vi "PCO_RecorderCopyAverageImage.vi"(0 "phRec":u64, 1 "wRoiX0":u16, 2 "wRoiX1":u16, 5 "phCam":u64, 7 "dwStartIdx":u32, 9 "dwStopIdx":u32, 11 "error in (no error)":errorcluster {"code" format="%x"}, 12 "wRoiY0":u16, 13 "wRoiY1":u16) -> (4 "phRec out":u64, 6 "ErrorMessage":i32 format="%x", 8 "wImgBuf":u16[][](array[numeric]), 15 "error out":errorcluster {"code" format="%x"})   [LabVIEW 2020, in "Recorder.lvlib"]
doc: "int WINAPI PCO_RecorderCopyAverageImage(HANDLE phRec, HANDLE phCam, DWORD dwStartIdx, DWORD dwStopIdx, WORD wRoiX0, WORD wRoiY0, WORD wRoiX1, WORD wRoiY1, WORD* wImgBuf);"
uses:
  Recorder.lvlib
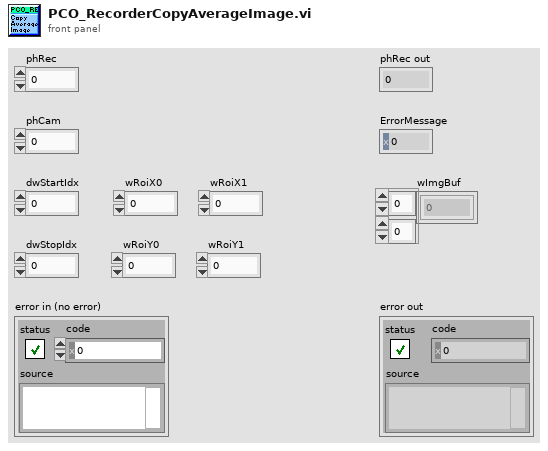
[diagram p1: front panel]
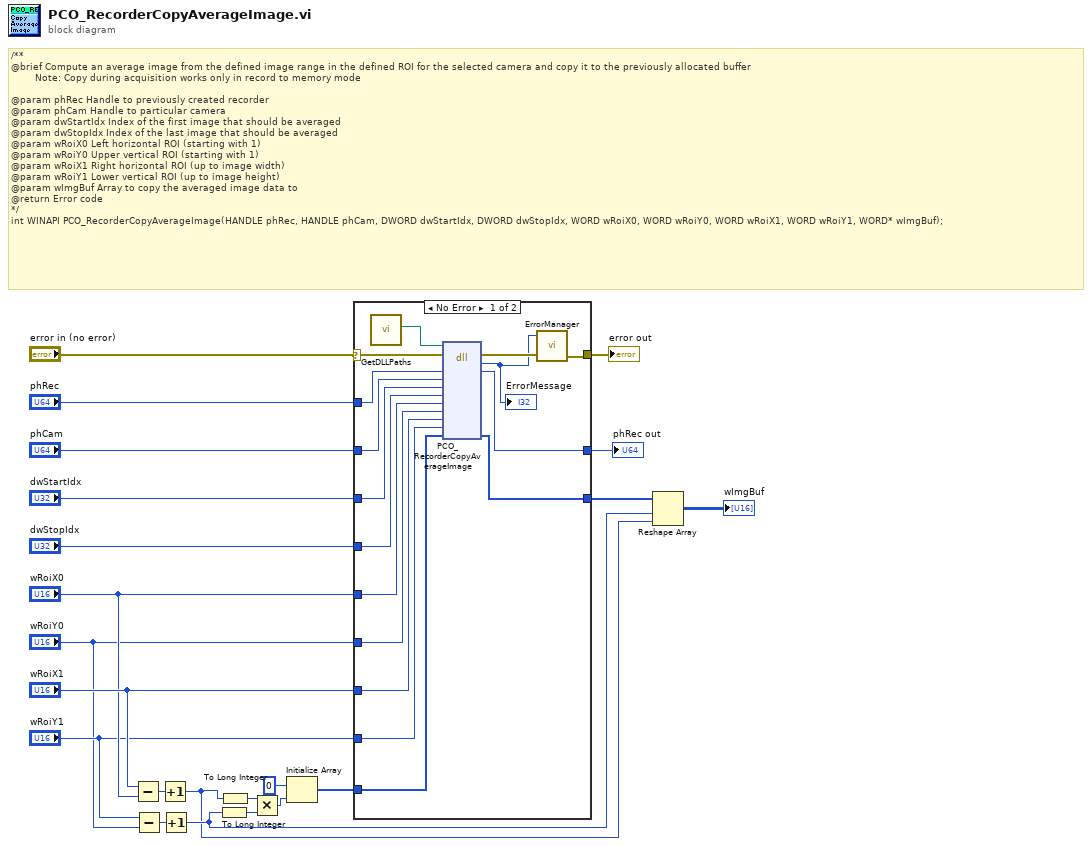
[diagram p0: block diagram]
diagram:
  # "/**\n@brief Compute an average image from the defined image range in the defined ROI for the selected camera and copy it to the previously allocated buffer\n        Note: Copy during acquisition works only in record to memory mode\n\n@param phRec Handle to previously created recorder\n@param phCam Handle to particular camera\n@param dwStartIdx Index of the first image that should be averaged\n@param dwStopIdx Index of the last image that should be averaged\n@param wRoiX0 Left horizontal ROI (starting with 1)\n@param wRoiY0 Upper vertical ROI (starting with 1)\n@param wRoiX1 Right horizontal ROI (up to image width)\n@param wRoiY1 Lower vertical ROI (up to image height)\n@param wImgBuf Array to copy the averaged image data to\n@return Error code\n*/\nint WINAPI PCO_RecorderCopyAverageImage(HANDLE phRec, HANDLE phCam, DWORD dwStartIdx, DWORD dwStopIdx, WORD wRoiX0, WORD wRoiY0, WORD wRoiX1, WORD wRoiY1, WORD* wImgBuf);"
  n1 = Subtract(x="wRoiX1", y="wRoiX0") -> (x-y=w11:u16)
  n2 = Subtract(x="wRoiY1", y="wRoiY0") -> (x-y=w10:u16)
  n3 = Increment(x=w11) -> (x+1=w2:u16)
  n4 = Increment(x=w10) -> (x+1=w3:u16)
  n5 = To Long Integer(number=w3) -> (32bit integer=w8:i32)
  n6 = To Long Integer(number=w2) -> (32bit integer=w7:i32)
  n7 = Multiply(x=w7, y=w8) -> (x*y=w9:i32)
  n8 = Initialize Array(u16 0 ("element"), w9) -> (w6:u16[])
  n9 = case shown="No Error" "error in (no error)" {
    selector: "error in (no error)" -> [w28 w41]
    tunnel: "phRec" -> [w38 w40]
    tunnel: [w37 w40] -> w21
    tunnel: "phCam" -> [w36 _]
    tunnel: "dwStartIdx" -> [w35 _]
    tunnel: "dwStopIdx" -> [w34 _]
    tunnel: [w33 w39] -> w4
    tunnel: [w25 w41] -> w17
    tunnel: "wRoiX1" -> [w32 _]
    tunnel: "wRoiX0" -> [w31 _]
    tunnel: "wRoiY1" -> [w30 _]
    tunnel: "wRoiY0" -> [w29 _]
    tunnel: w6 -> [w27 w39]
    frame No Error {
      n10 = call "GetDLLPaths.vi"() -> ("PCO_Recorder_Path"=w23:path)  [unwired: 9 in, 2 out]
      n11 = dll-call lib="?" fn="PCO_RecorderCopyAverageImage"(path in=w23, error in=w28, "phRec"=w38, "phCam"=w36, "dwStartIdx"=w35, "dwStopIdx"=w34, "wRoiX0"=w31, "wRoiY0"=w29, "wRoiX1"=w32, "wRoiY1"=w30, "wImgBuf"=w27) -> (error out=w26:errorcluster, "return type"=w24:i32, "phRec"=w37:u64, "wImgBuf"=w33:u16[])  [unwired: 8 in, 1 out]
      "ErrorMessage" <- w24
      n12 = call "ErrorManager.vi"("error in (no error)"=w26, "error code"=w24) -> ("error out"=w25:errorcluster)  [unwired: 3 in]
    }
    frame Error {
    }
  }
  "phRec out" <- w21
  "error out" <- w17
  n13 = Reshape Array(w4, w3, w2) -> (→"wImgBuf":u16[][])
